vi "JX_MoveBySteps.vi"(6 "Direction":bool, 7 "Channel":u8, 8 "error in (no error)":errorcluster, 9 "CH0 Steps/deg":u16, 11 "MB_Master in":refnum<class "MB_Master.lvclass">=refnum) -> (0 "error out":errorcluster, 3 "MB_Master out":refnum<class "MB_Master.lvclass">)   [LabVIEW 2023]
uses:
  <vilib>/Plasmionique/MB Master/MB_Master/MB_Master.lvclass
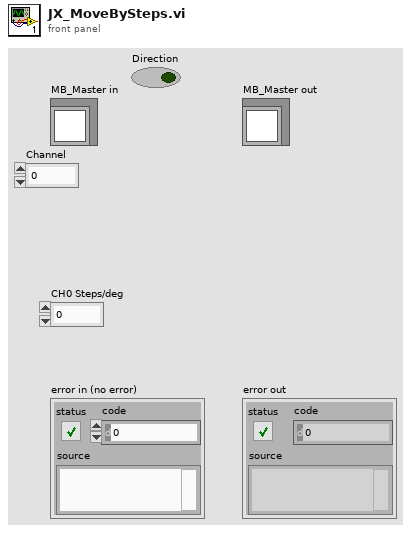
[diagram p1: front panel]
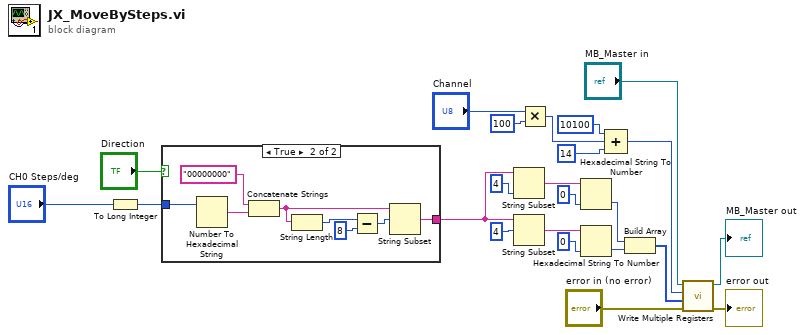
[diagram p0: block diagram]
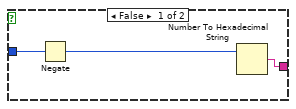
[diagram p2: hidden frame]
diagram:
  n1 = To Long Integer(number="CH0 Steps/deg") -> (32bit integer=w2:i32)
  n2 = case shown="True" "Direction" {
    tunnel: [w24 w29] -> w3
    tunnel: w2 -> [w25 w28]
    frame False {
      n3 = Negate(x=w25) -> (-x=w26:i32)
      n4 = Number To Hexadecimal String(2:w26) -> (0:w24:string)  [unwired: 1 in]
    }
    frame True {
      n5 = Number To Hexadecimal String(2:w28) -> (0:w27:string)  [unwired: 1 in]
      n6 = Concatenate Strings("00000000", w27) -> (w34:string)
      n7 = String Length(string=w34) -> (length=w33:i32)
      n8 = Subtract(x=w33, y=8) -> (x-y=w31:i32)
      n9 = String Subset(string=w34, offset (0)=w31) -> (substring=w29:string)  [unwired: 1 in]
    }
  }
  n10 = String Subset(string=w3, length (rest)=4 ("length (rest)")) -> (substring=w17:string)  [unwired: 1 in]
  n11 = String Subset(string=w3, offset (0)=4) -> (substring=w19:string)  [unwired: 1 in]
  n12 = Multiply(x="Channel", y=u16 100) -> (x*y=w10:u16)
  n13 = Hexadecimal String To Number(string=w17, default (0uL)=u16 0 ("default (0 U32)")) -> (number=w21:u16)  [unwired: 1 in, 1 out]
  n14 = Hexadecimal String To Number(string=w19, default (0uL)=u16 0 ("default (0 U32)")) -> (number=w22:u16)  [unwired: 1 in, 1 out]
  n15 = Compound Arithmetic op=ADD(u16 10100 ("value"), w10, u8 14 ("value")) -> (w5:u16)
  n16 = Build Array(w21, w22) -> (w12:u16[])
  n17 = call <vilib>:"Write Multiple Registers.vi"("error in (no error)"="error in (no error)", "values"=w12, "starting address"=w5, "MB session in"="MB_Master in") -> ("error out"=→"error out":errorcluster, "MB session out"=→"MB_Master out":refnum<class "MB_Master.lvclass">)  [unwired: 6 in]
